vi "Load External Modules.vi"(8 "error in (no error)":errorcluster, 11 "Application Controller in":refnum<class "Application Controller.lvclass">) -> (0 "error out":errorcluster, 3 "Application Controller out":refnum<class "Application Controller.lvclass">)   [LabVIEW 2016, in "Application Controller.lvclass"]
uses:
  Application Controller.lvclass
  Application Controller.lvclass/Application Controller.ctl
  Template Module/Template Module.lvclass/Template Module.ctl
  Template Module/Read Name.vi
  Read Startup Configuration.vi
  Read Start-up configuration file.vi
  Template Module/Template Module.lvclass
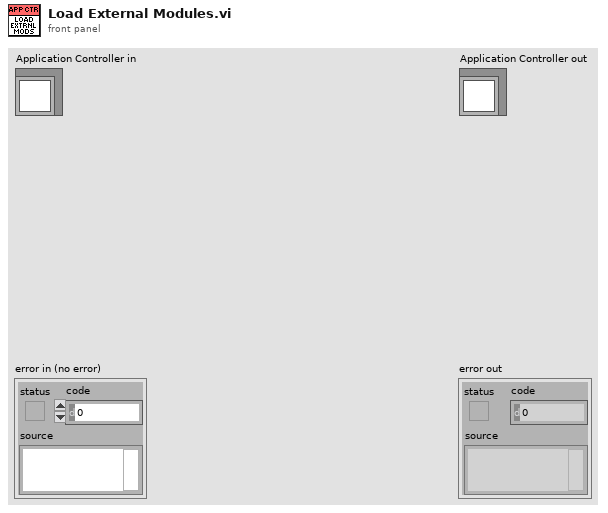
[diagram p1: front panel]
types:
  T1 = typedef "Start-up Configuration.ctl" = cluster{"Load Modules":T2[], "External Modules Loaders":string[]}
  T2 = typedef "Module Types.ctl" = enum16{"NONE", "NI-DAQmx", "NI-Scope", "Red Pitaya Digitizer", "GaGe", "VISA Device", "Red Pitaya Lockin", "Monitor Controller", "Pulse Controller", "Integrate Pulse", "Lockin Processor", "File converter", "NHMFL Synthesizer", "Micron Hyperion", "Spectrum Recorder", "Resonance Detector", "TCP Communications", "Format Resonances", "Ruby Spectra", "PID Controller"}
  T3 = typedef "Menu Control.ctl" = enum16{"NONE", "Monitor", "Post-process", "Pulse"}
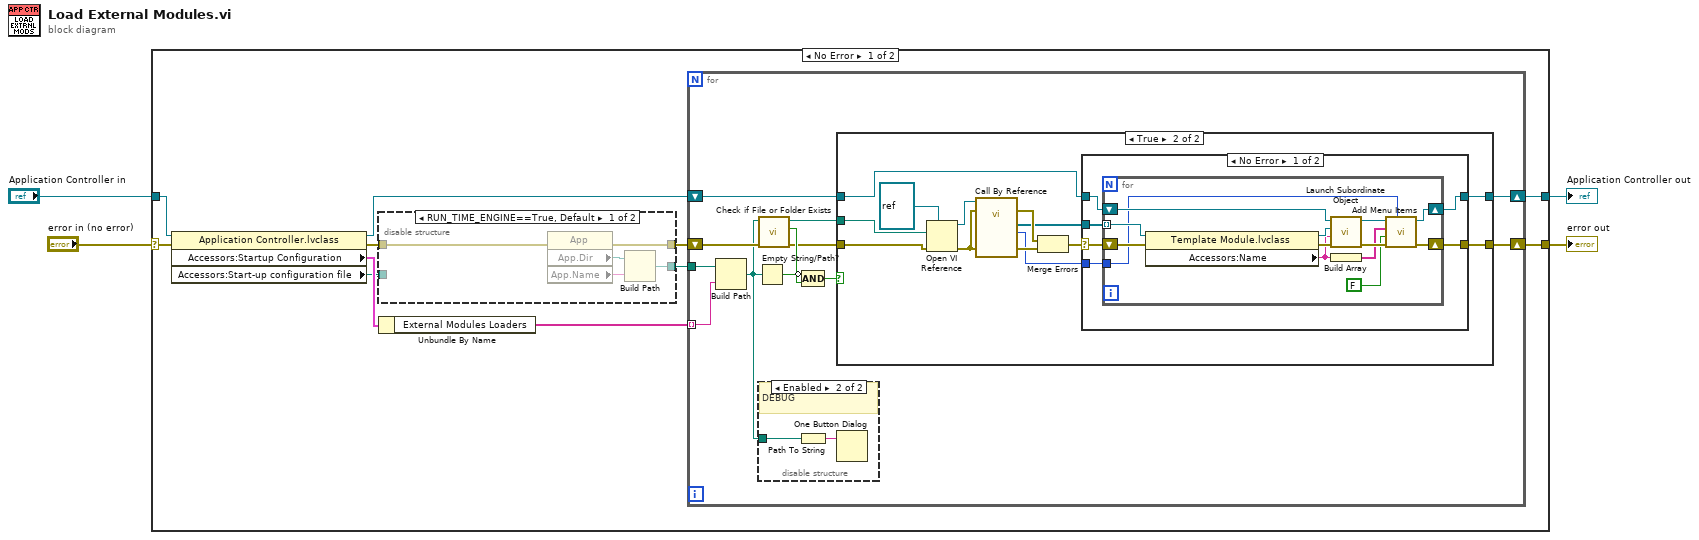
[diagram p0: block diagram]
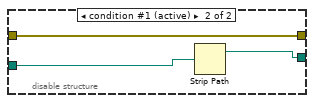
[diagram p2: hidden frame]
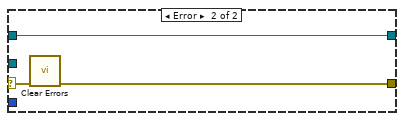
[diagram p5: hidden frame]
diagram:
  n1 = case shown="No Error" "error in (no error)" {
    selector: "error in (no error)" -> [w15 w76]
    tunnel: [w11 w76] -> w3
    tunnel: [w9 w75] -> w1
    tunnel: "Application Controller in" -> [w14 w75]
    frame No Error {
      n2 = property class="Application Controller.lvclass"(reference=w14, error in=w15) -> (reference out=w10:refnum<class "Application Controller.lvclass">, error out=w6:errorcluster, "Accessors:Startup Configuration"=w13:T1, "Accessors:Start-up configuration file"=w8:path)
      n3 = disable-structure shown="RUN_TIME_ENGINE==True, Default" {
        disable-tunnel: w8 -> [_ w23]
        disable-tunnel: [w16 w22] -> w7
        disable-tunnel: w6 -> [w20 w21]
        disable-tunnel: [w19 w21] -> w5
        frame condition #0 {
          n4 = property class="App"(error in=w20) -> (error out=w19:errorcluster, "App.Dir"=w18:path, "App.Name"=w17:string)  [unwired: 1 in, 1 out]
          n5 = Build Path(base path=w18, name or relative path=w17) -> (appended path=w16:path)
        }
        frame condition #1 (active) {
          n6 = Strip Path(path=w23) -> (stripped path=w22:path)  [unwired: 1 out]
        }
      }
      n7 = Unbundle By Name(w13) -> ("External Modules Loaders"=w12:string[])
      n8 = for {
        tunnel: w12 -> [w25] mode=indexing
        shift-right: [w28] -> w11
        shift-left: w5 -> [w33]
        shift-right: [w27] -> w9
        shift-left: w10 -> [w29]
        tunnel: w7 -> [w26]
        n9 = Build Path(base path=w26, name or relative path=w25) -> (appended path=w24:path)
        n10 = Empty String/Path?(string/path=w24) -> (empty?=w35:bool)
        n11 = call <vilib>:"Check if File or Folder Exists.vi"("error in (no error)"=w33, "path"=w24) -> ("error out"=w31:errorcluster, "file or folder exists?"=w34:bool, "dup path"=w30:path)  [unwired: 7 in]
        n12 = disable-structure shown="Enabled" {
          disable-tunnel: w24 -> [_ w37]
          frame Disabled {
          }
          frame Enabled {
            # "DEBUG"
            n13 = Path To String(path=w37) -> (string=w36:string)
            n14 = One Button Dialog(message=w36) -> ()  [unwired: 1 in, 1 out]
          }
        }
        n15 = Compound Arithmetic op=AND(invert w35, w34) -> (w32:bool)
        n16 = case shown="True" w32 {
          tunnel: w31 -> [w39 w50]
          tunnel: w30 -> [_ w49]
          tunnel: w29 -> [w38 w44]
          tunnel: [w39 w42] -> w28
          tunnel: [w38 w41] -> w27
          frame False {
          }
          frame True {
            n17 = Open VI Reference(type specifier VI Refnum (for type only)=refnum<vi> refnum, vi path=w49, error in (no error)=w50) -> (vi reference=w52:refnum<vi>, error out=w48:errorcluster)  [unwired: 3 in]
            n18 = call-by-ref "?"(reference=w52, error in=w48, "Error In"=w48) -> (error out=w47:errorcluster, "Error Out"=w46:errorcluster, "Menu control"=w40:T3, "Modules"=w43:refnum<class "Template Module.lvclass">[])  [unwired: 8 in, 1 out]
            n19 = Merge Errors(w47, w46) -> (w45:errorcluster)
            n20 = case shown="No Error" w45 {
              selector: w45 -> [w57 w74]
              tunnel: w44 -> [w56 w72]
              tunnel: w43 -> [w58 _]
              tunnel: [w55 w73] -> w42
              tunnel: [w54 w72] -> w41
              tunnel: w40 -> [w53 _]
              frame No Error {
                n21 = for {
                  tunnel: w58 -> [w71] mode=indexing
                  shift-right: [w60] -> w54
                  shift-left: w56 -> [w67]
                  shift-right: [w61] -> w55
                  shift-left: w57 -> [w70]
                  tunnel: w53 -> [w59]
                  n22 = property class="Template Module.lvclass"(reference=w71, error in=w70) -> (reference out=w68:refnum<class "Template Module.lvclass">, error out=w69:errorcluster, "Accessors:Name"=w64:string)
                  n23 = call-dynamic "Launch Subordinate Object.vi"("error in (no error)"=w69, "Name"=w64, "Subordinate Object"=w68, "Measure Object in"=w67) -> ("error out"=w65:errorcluster, "Measure Object out"=w66:refnum<class "Application Controller.lvclass">)  [unwired: 5 in, 1 out]
                  n24 = Build Array(w64) -> (w63:string[])
                  n25 = call-dynamic "Add Menu Items.vi"("Menu control"=w59, "error in (no error)"=w65, "Reset"=FALSE, "Item Names"=w63, "Monitor-Pulse in"=w66) -> ("error out"=w61:errorcluster, "Monitor-Pulse out"=w60:refnum<class "Application Controller.lvclass">)  [unwired: 5 in]
                }
              }
              frame Error {
                n26 = call <vilib>:"Clear Errors.vi"("error in (no error)"=w74) -> ("error out"=w73:errorcluster)  [unwired: 5 in, 1 out]
              }
            }
          }
        }
      }
    }
    frame Error {
    }
  }
  "error out" <- w3
  "Application Controller out" <- w1
